vi "Insert_subvi_to_subpanel.vi"(5 "SubVI path":path, 6 "HART resource name":refnum<visa-resource-name>="HART", 7 "subpanel ref":refnum<vi>, 8 "Input number":i32, 9 "MODBUS resource name":refnum<visa-resource-name>="485", 10 "Index":u16(ring) items=["None", "Pulse Input", "Current Input", "Serial Input"], 11 "Array of VIs to insert":string[](array[string])) -> (0 "error out":errorcluster, 3 "VI reference out":refnum<vi>)   [LabVIEW 2016]
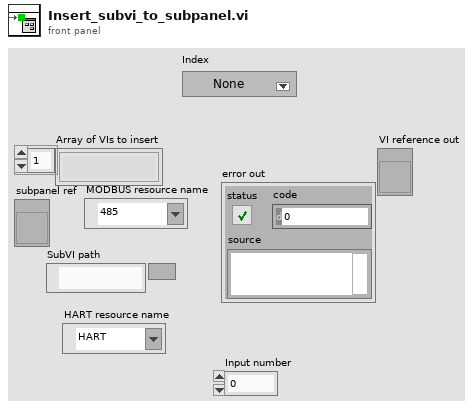
[diagram p1: front panel]
types:
  T1 = enum16{"Always On", "Always Off", "Off While Running"}
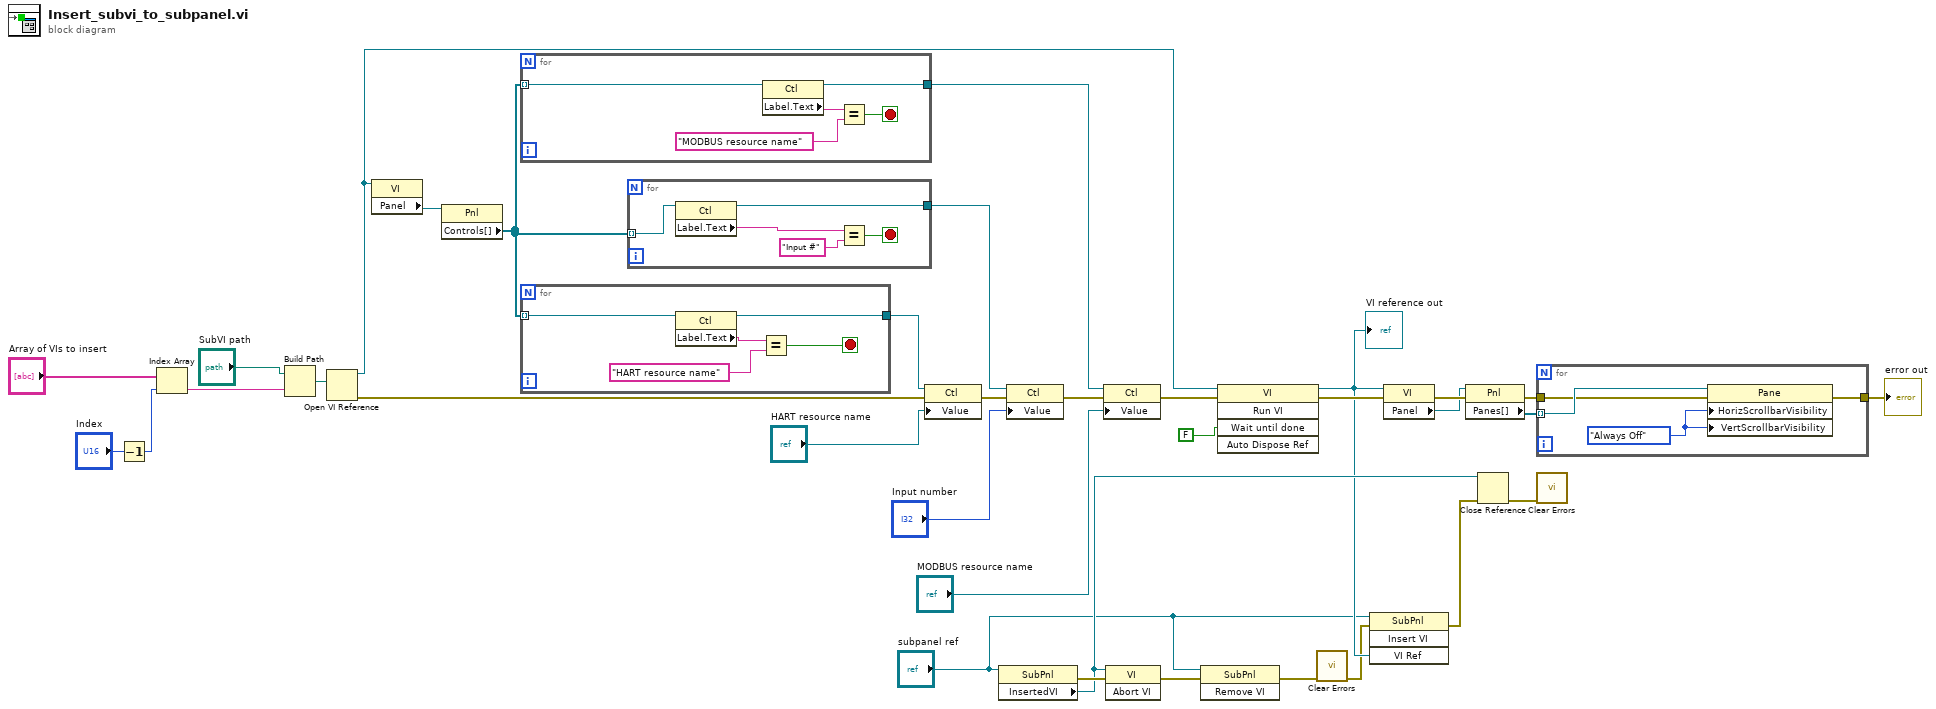
[diagram p0: block diagram]
diagram:
  n1 = Decrement(x="Index") -> (x-1=w25:u16)
  n2 = Index Array(array="Array of VIs to insert", index=w25) -> (element=w32:string)
  n3 = Build Path(base path="SubVI path", name or relative path=w32) -> (appended path=w33:path)
  n4 = Open VI Reference(vi path=w33) -> (vi reference=w16:refnum<vi>, error out=w6:errorcluster)  [unwired: 5 in]
  n5 = property class="VI"(reference=w16) -> ("Panel"=w18:refnum<vi>)  [unwired: 1 in, 2 out]
  n6 = property class="Pnl"(reference=w18) -> ("Controls[]"=w4:refnum<vi>[])  [unwired: 1 in, 2 out]
  n7 = for {
    tunnel: w4 -> [w36] mode=indexing
    tunnel: [w37] -> w19
    stop <- w38 stop-if-true
    n8 = property class="Ctl"(reference=w36) -> (reference out=w37:refnum<vi>, "Label.Text"=w40:string)  [unwired: 1 in, 1 out]
    n9 = Equal?(x=w40, y="MODBUS resource name") -> (x = y?=w38:bool)
  }
  n10 = for {
    tunnel: w4 -> [w41] mode=indexing
    tunnel: [w42] -> w8
    stop <- w43 stop-if-true
    n11 = property class="Ctl"(reference=w41) -> (reference out=w42:refnum<vi>, "Label.Text"=w45:string)  [unwired: 1 in, 1 out]
    n12 = Equal?(x=w45, y="HART resource name") -> (x = y?=w43:bool)
  }
  n13 = for {
    tunnel: w4 -> [w46] mode=indexing
    tunnel: [w47] -> w5
    stop <- w48 stop-if-true
    n14 = property class="Ctl"(reference=w46) -> (reference out=w47:refnum<vi>, "Label.Text"=w50:string)  [unwired: 1 in, 1 out]
    n15 = Equal?(x=w50, y="Input #") -> (x = y?=w48:bool)
  }
  n16 = property class="Ctl"(reference=w8, error in=w6, "Value"="HART resource name") -> (error out=w3:errorcluster)  [unwired: 1 out]
  n17 = property class="SubPnl"(reference="subpanel ref") -> (error out=w31:errorcluster, "InsertedVI"=w29:refnum<vi>)  [unwired: 1 in, 1 out]
  n18 = property class="Ctl"(reference=w5, error in=w3, "Value"="Input number") -> (error out=w2:errorcluster)  [unwired: 1 out]
  n19 = property class="Ctl"(reference=w19, error in=w2, "Value"="MODBUS resource name") -> (error out=w17:errorcluster)  [unwired: 1 out]
  n20 = invoke class="VI" method="Abort VI"(reference=w29, error in=w31) -> (error out=w28:errorcluster)  [unwired: 1 in, 2 out]
  n21 = invoke class="SubPnl" method="Remove VI"(reference="subpanel ref", error in=w28) -> (error out=w27:errorcluster)  [unwired: 1 in, 2 out]
  n22 = invoke class="VI" method="Run VI"(reference=w16, error in=w17, "Wait until done"=FALSE ("Wait Until Done")) -> (reference out=w20:refnum<vi>, error out=w24:errorcluster)  [unwired: 2 in, 3 out]
  "VI reference out" <- w20
  n23 = call <vilib>:"Clear Errors.vi"("error in (no error)"=w27) -> ("error out"=w15:errorcluster)  [unwired: 5 in, 1 out]
  n24 = invoke class="SubPnl" method="Insert VI"(reference="subpanel ref", error in=w15, "VI Ref"=w20) -> (error out=w30:errorcluster)  [unwired: 1 in, 3 out]
  n25 = property class="VI"(reference=w20, error in=w24) -> (error out=w23:errorcluster, "Panel"=w21:refnum<vi>)  [unwired: 1 out]
  n26 = property class="Pnl"(reference=w21, error in=w23) -> (error out=w22:errorcluster, "Panes[]"=w35:refnum<vi>[])  [unwired: 1 out]
  n27 = Close Reference(reference=w29, error in (no error)=w30) -> (error out=w26:errorcluster)
  n28 = for {
    tunnel: w35 -> [w54] mode=indexing
    tunnel: w22 -> [w52]
    tunnel: [w51] -> w10
    w53 = T1."Always Off" ("Horizontal Scrollbar Visibility")
    n29 = property class="Pane"(reference=w54, error in=w52, "HorizScrollbarVisibility"=w53, "VertScrollbarVisibility"=w53) -> (error out=w51:errorcluster)  [unwired: 1 out]
  }
  "error out" <- w10
  n30 = call <vilib>:"Clear Errors.vi"("error in (no error)"=w26) -> ()  [unwired: 5 in, 2 out]
